vi "swerve_forwards_kinematics.vi"(1 "Input Vector":T1) -> (0 "Output Vector":T1)   [LabVIEW 2020]
uses:
  <vilib>/Analysis/Matrix/Datatypes/RealMatrix.ctl
  <vilib>/Analysis/_algsub.llb/Real PseudoInverse Matrix.vi
  <vilib>/Analysis/Matrix/Numeric/Conversions/Array To Matrix - RA2.vi
  <vilib>/Analysis/Matrix/Numeric/Multiply/Multiply - RM,RM.vi
  <vilib>/Analysis/Matrix/NI_Matrix.lvlib
  <vilib>/Analysis/NI_AALPro.lvlib
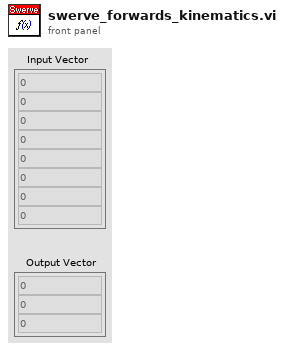
[diagram p1: front panel]
types:
  T1 = typedef "NI_Matrix.lvlib/RealMatrix.ctl" = dbl[][]
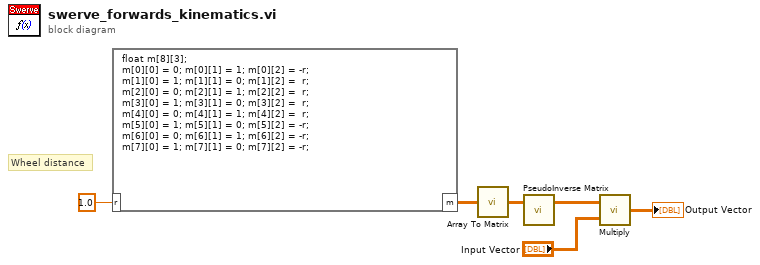
[diagram p0: block diagram]
diagram:
  # "Wheel distance"
  n1 = formula code="float m[8][3];\nm[0][0] = 0; m[0][1] = 1; m[0][2] = -r;\nm[1][0] = 1; m[1][1] = 0; m[1][2] =  r;\nm[2][0] = 0; m[2][1] = 1; m[2][2] =  r;\nm[3][0] = 1; m[3][1] = 0; m[3][2] =  r;\nm[4][0] = 0; m[4][1] = 1; m[4][2] =  r;\nm[5][0] = 1; m[5][1] = 0; m[5][2] = -r;\nm[6][0] = 0; m[6][1] = 1; m[6][2] = -r;\nm[7][0] = 1; m[7][1] = 0; m[7][2] = -r;"("r"=1.0 ("input variable")) -> ("m"=w6:dbl[][])
  n2 = call-poly <vilib>:"Array To Matrix.vi"("Real 2D Array"=w6) -> ("Real Matrix"=w5:T1)
  n3 = call-poly <vilib>:"PseudoInverse Matrix.vi"("Input Matrix"=w5) -> ("PseudoInverse Matrix"=w4:T1)  [unwired: 1 in, 1 out]
  n4 = call-poly <vilib>:"Multiply.vi"("Real Matrix B"="Input Vector", "Real Matrix A"=w4) -> ("A * B"=→"Output Vector":T1)
